vi "pre_processamento.vi"() -> ()   [LabVIEW 2020]
uses:
  <vilib>/numeric/Random Number (Range) DBL.vi
panel:
  out "result 3":dbl[](array[numeric])
  out "Array 6":dbl[](array[numeric])
  out "Array 5":dbl[](array[numeric])
  out "number 3":dbl
  out "Multiplicação A 3":dbl[](graph)
  out "result 2":dbl[](array[numeric])
  out "Array 4":dbl[](array[numeric])
  out "Array 3":dbl[](array[numeric])
  out "number 2":dbl
  out "Multiplicação A 2":dbl[](graph)
  out "result":dbl[](array[numeric])
  out "Array 2":dbl[](array[numeric])
  out "Array":dbl[](array[numeric])
  out "number":dbl
  out "Corrente da Fase A":dbl[](graph)
  out "Tensão da Fase A":dbl[](graph)
  out "Multiplicação A":dbl[](graph)
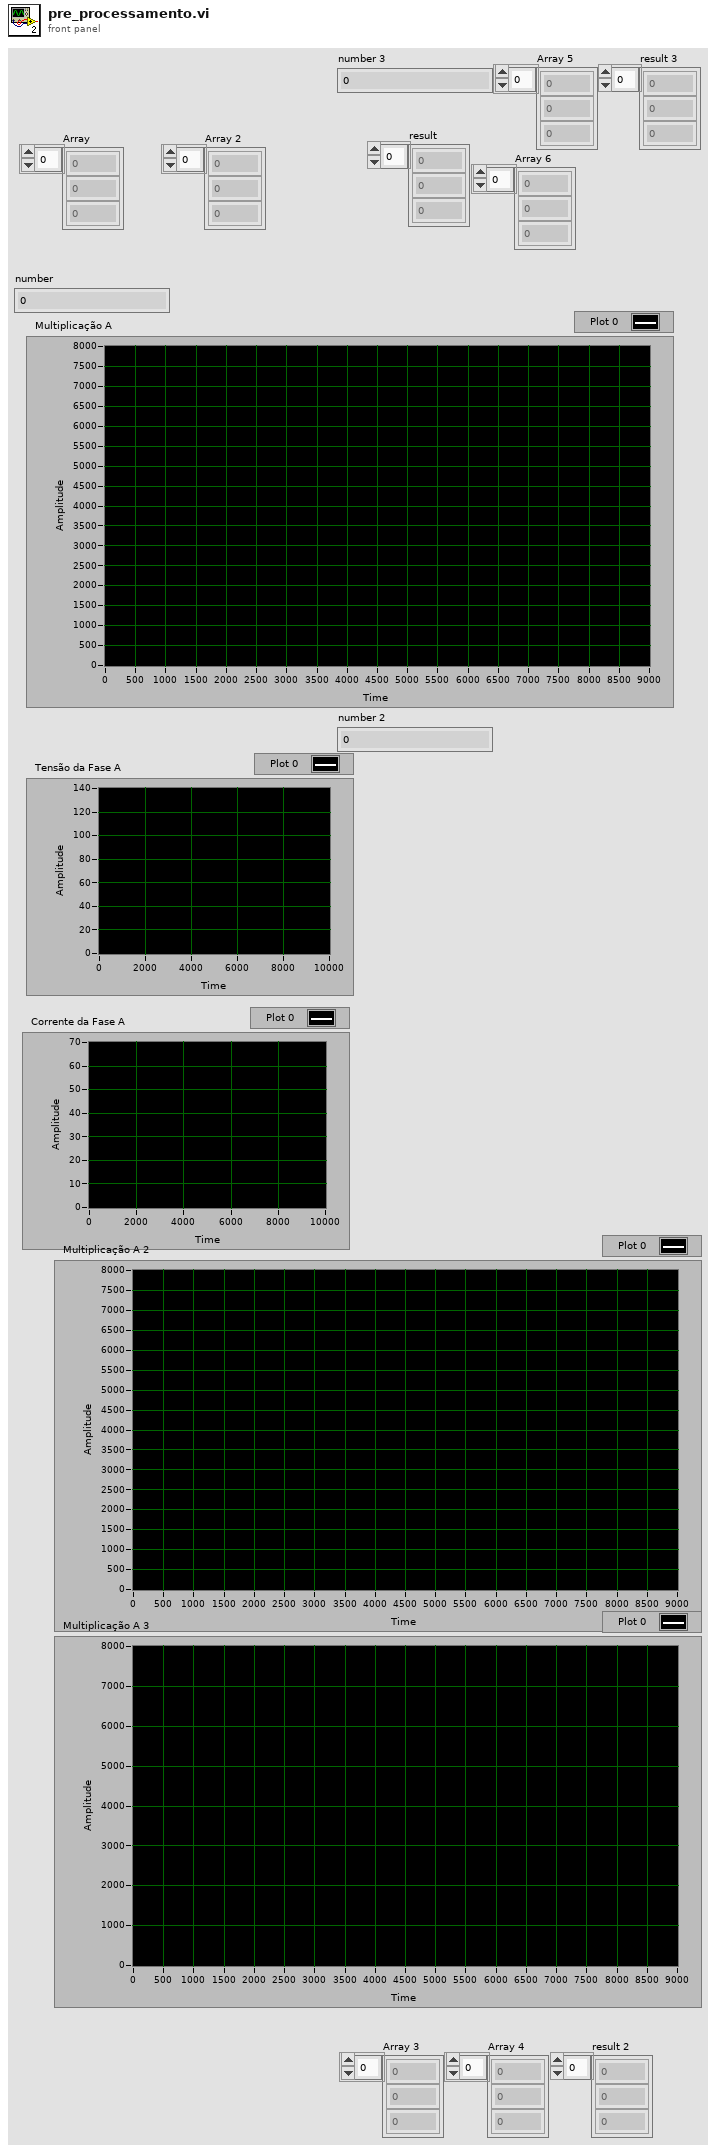
[diagram p1: front panel]
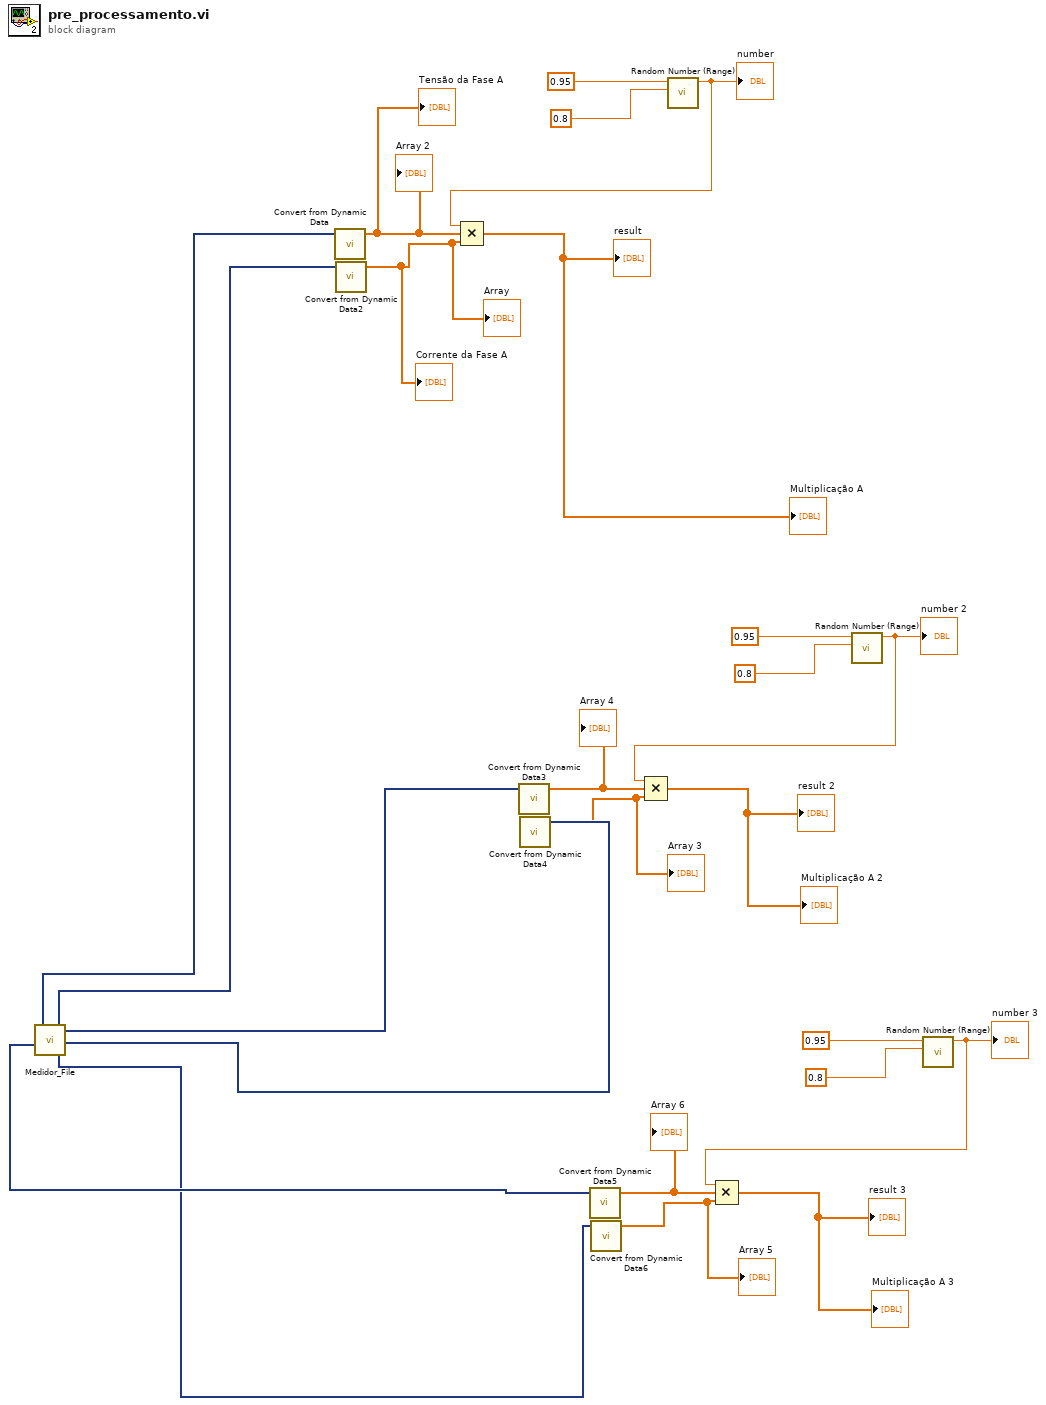
[diagram p0: block diagram]
diagram:
  n1 = call "Medidor_File.vi"() -> ("Corrente Fase C"=w2:dynamicdata, "Corrente Fase B"=w11:dynamicdata, "Corrente Fase A"=w24:dynamicdata, "Tensão Fase C"=w3:dynamicdata, "Tensão Fase B"=w12:dynamicdata, "Tensão Fase A"=w23:dynamicdata)  [unwired: 1 out]
  n2 = call "Convert from Dynamic Data"("Dynamic Data Type"=w23) -> ("Array"=w19:dbl[])  [unwired: 3 in]
  "Tensão da Fase A" <- w19
  "Array 2" <- w19
  n3 = call "Convert from Dynamic Data2"("Dynamic Data Type"=w24) -> ("Array"=w1:dbl[])  [unwired: 3 in]
  "Corrente da Fase A" <- w1
  "Array" <- w1
  n4 = call "Convert from Dynamic Data3"("Dynamic Data Type"=w12) -> ("Array"=w14:dbl[])  [unwired: 3 in]
  "Array 4" <- w14
  n5 = call "Convert from Dynamic Data4"("Dynamic Data Type"=w11) -> ("Array"=w10:dbl[])  [unwired: 3 in]
  "Array 3" <- w10
  n6 = call "Convert from Dynamic Data5"("Dynamic Data Type"=w3) -> ("Array"=w6:dbl[])  [unwired: 3 in]
  "Array 6" <- w6
  n7 = call "Convert from Dynamic Data6"("Dynamic Data Type"=w2) -> ("Array"=w4:dbl[])  [unwired: 3 in]
  "Array 5" <- w4
  n8 = call-poly <vilib>:"Random Number (Range).vi"("lower bound (0)"=0.8, "upper bound (100)"=0.95) -> ("number"=w20:dbl)  [unwired: 9 in]
  "number" <- w20
  n9 = Compound Arithmetic op=MULTIPLY(w20, w19, w1) -> (→"Multiplicação A" →"result":dbl[])
  n10 = call-poly <vilib>:"Random Number (Range).vi"("lower bound (0)"=0.8, "upper bound (100)"=0.95) -> ("number"=w15:dbl)  [unwired: 9 in]
  "number 2" <- w15
  n11 = Compound Arithmetic op=MULTIPLY(w15, w14, w10) -> (→"Multiplicação A 2" →"result 2":dbl[])
  n12 = call-poly <vilib>:"Random Number (Range).vi"("lower bound (0)"=0.8, "upper bound (100)"=0.95) -> ("number"=w7:dbl)  [unwired: 9 in]
  "number 3" <- w7
  n13 = Compound Arithmetic op=MULTIPLY(w7, w6, w4) -> (→"Multiplicação A 3" →"result 3":dbl[])
